vi "Read Transformation matrix.vi"(8 "error in (no error)":errorcluster, 11 "Transform in":refnum<class "Transform.lvclass">) -> (0 "error out":errorcluster, 2 "Transformation matrix":dbl[][](array[numeric]), 3 "Transform out":refnum<class "Transform.lvclass">)   [LabVIEW 2013, in "MaterialCharacterization.lvlib" / "Transform.lvclass"]
uses:
  Transform.lvclass
  Transform.lvclass/Transform.ctl
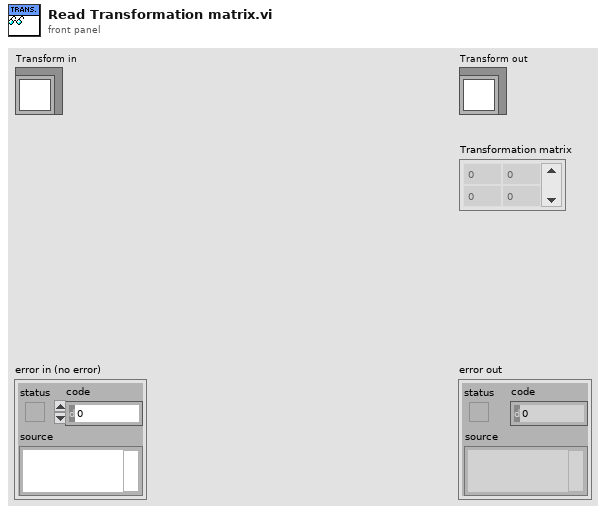
[diagram p1: front panel]
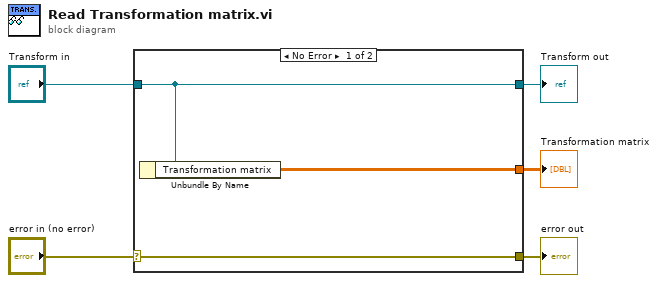
[diagram p0: block diagram]
diagram:
  n1 = case shown="No Error" "error in (no error)" {
    selector: "error in (no error)" -> [w8 w9]
    tunnel: [w8 w9] -> w4
    tunnel: [w7 w10] -> w2
    tunnel: "Transform in" -> [w7 w10]
    tunnel: [w6 _] -> w1
    frame No Error {
      n2 = Unbundle By Name(w7) -> ("Transformation matrix"=w6:dbl[][])
    }
    frame Error {
    }
  }
  "error out" <- w4
  "Transform out" <- w2
  "Transformation matrix" <- w1
